vi "Is Active.vi"(10 "cycle count":u64=1, 11 "Plugin in":refnum<class "Plugin.lvclass">) -> (2 "active this cycle?":bool, 3 "Plugin out":refnum<class "Plugin.lvclass">)   [LabVIEW 2019, in "DSF Core.lvlib" / "Plugin.lvclass"]
uses:
  Plugin.lvclass
  Plugin.lvclass/Plugin.ctl
  Timing/Timing.lvclass/Timing.ctl
  Timing/Get Decimation.vi
  Timing/Get Offset.vi
  Timing/Timing.lvclass
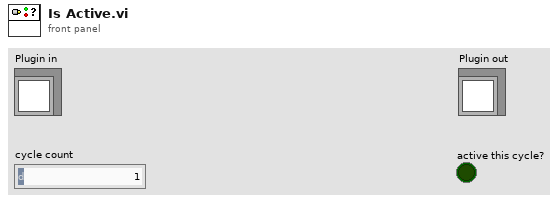
[diagram p1: front panel]
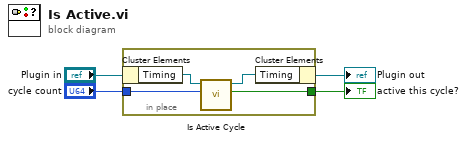
[diagram p0: block diagram]
diagram:
  n1 = in-place {
    in-place-border: "cycle count" -> [w8]
    in-place-border: [w7] -> w3
    n2 = in-place-cluster #1("Plugin in") -> ("Timing"=w6:refnum<class "Timing.lvclass">)
    n3 = call "Is Active Cycle.vi"("iteration"=w8, "Timing in"=w6) -> ("active?"=w7:bool, "Timing out"=w5:refnum<class "Timing.lvclass">)  [unwired: 8 in]
    n4 = in-place-cluster #1("Timing"=w5) -> (→"Plugin out":refnum<class "Plugin.lvclass">)
  }
  "active this cycle?" <- w3
